vi "InitVolumeAndTimeSamples.vi"   [LabVIEW 2013]
uses:
  GlobalVariables/VolumeAndTimeSamplesvi.vi
types:
  T1 = cluster{"TimeSamples":dbl[], "VolumeSamples":dbl[]}
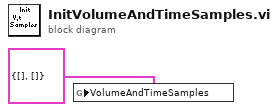
[diagram p0: block diagram]
diagram:
  n1 = global write "VolumeAndTimeSamplesvi.vi" "VolumeAndTimeSamples"(T1 {"TimeSamples"=[], "VolumeSamples"=[]} ("VolumeAndTimeSamples")) -> ()
